vi "get_range_table_cmd_value.vi"(7 "Range Table ID in":string, 8 "error in":errorcluster caption="error in (no error)", 10 "Input Int32 value":i32 caption="I32 input", 11 "VISA resource name":refnum<visa-resource-name>) -> (0 "error out":errorcluster, 2 "Cmd value out":string caption="String Value out", 3 "VISA resource name out":refnum<visa-resource-name>)   [LabVIEW 2020, in "Rohde&Schwarz RTx Oscilloscopes.lvlib" / "rsidr_core.lvlib"]
doc: "Only works with Discrete Range Tables - convers the input Int32 value to an output command string.\nFor other range table types converts int32 to string as a number."
uses:
  rsidr_core.lvlib
  _type_Operation_Fgv_RangeTable.ctl
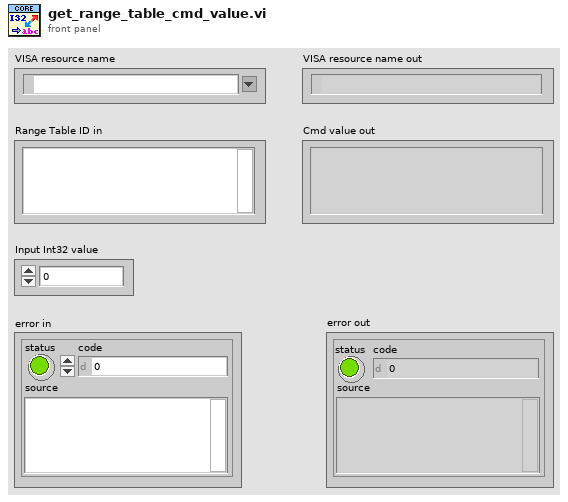
[diagram p1: front panel]
types:
  T1 = typedef "Rohde&Schwarz RTx Oscilloscopes.lvlib/rsidr_core.lvlib/_type_Operation_Fgv_RangeTable.ctl" = enum16{"Initialize", "Check", "Coerce", "Get Command String", "Get Numeric Value", "Get Default Value", "Get Range Table Type"}
  T2 = typedef "Rohde&Schwarz RTx Oscilloscopes.lvlib/rsidr_core.lvlib/_type_RangeTable_Type.ctl" = enum16{"Ranged", "Coerced", "Discrete"}
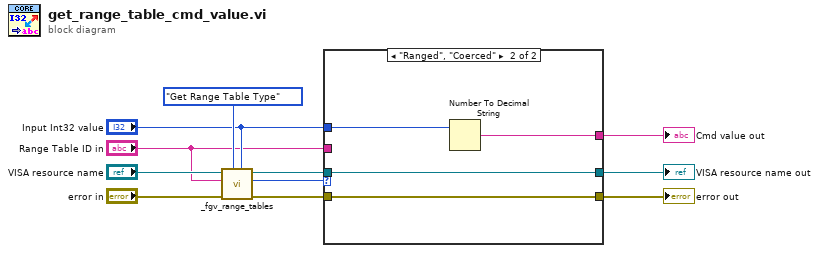
[diagram p0: block diagram]
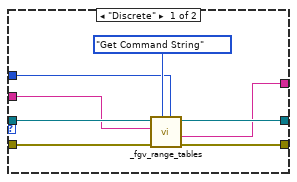
[diagram p2: hidden frame]
diagram:
  n1 = call "_fgv_range_tables.vi"("Numeric Value in (0.0)"="Input Int32 value", "Operation"=_type_Operation_Fgv_RangeTable."Get Range Table Type", "error in"="error in", "Range Table ID in"="Range Table ID in", "VISA resource name"="VISA resource name") -> ("error out"=w5:errorcluster, "Range Table Type out"=w8:T2, "VISA resource name out"=w4:refnum<visa-resource-name>)  [unwired: 2 in, 2 out]
  n2 = case shown="\"Ranged\", \"Coerced\"" w8 {
    tunnel: "Input Int32 value" -> [w13 w23]
    tunnel: [w15 w22] -> w6
    tunnel: w5 -> [w19 w20]
    tunnel: w4 -> [w18 w21]
    tunnel: [w17 w20] -> w3
    tunnel: [w16 w21] -> w2
    tunnel: "Range Table ID in" -> [w12 _]
    frame "Discrete" {
      n3 = call "_fgv_range_tables.vi"("Numeric Value in (0.0)"=w13, "Operation"=_type_Operation_Fgv_RangeTable."Get Command String", "error in"=w19, "Range Table ID in"=w12, "VISA resource name"=w18) -> ("error out"=w17:errorcluster, "String Value out"=w15:string, "VISA resource name out"=w16:refnum<visa-resource-name>)  [unwired: 2 in, 2 out]
    }
    frame "Ranged", "Coerced" {
      n4 = Number To Decimal String(number=w23) -> (decimal integer string=w22:string)  [unwired: 1 in]
    }
  }
  "VISA resource name out" <- w2
  "error out" <- w3
  "Cmd value out" <- w6
